vi "Sort_AI_Data.vi"(7 "Inclin":T3, 10 "AI_data":dbl[](array[numeric]), 11 "AlarmSettings":T1={"TC13"={"Enbl"=FALSE, "ErrsAndWarns"={0.0, 5.663716814159292, 7.168141592920354, 8.584070796460177}}, "AI1"={"Enbl"=FALSE, "ErrsAndWarns"={0.0, 5.663716814159292, 7.168141592920354, 8.584070796460177}}, "AI2"={"Enbl"=FALSE, "ErrsAndWarns"={0.0, 5.663716814159292, 7.168141592920354, 8.584070796460177}}, "AI3"={"Enbl"=FALSE, "ErrsAndWarns"={0.0, 5.663716814159292, 7.168141592920354, 8.584070796460177}}, "AI4"={"Enbl"=FALSE, "ErrsAndWarns"={0.0, 5.663716814159292, 7.168141592920354, 8.584070796460177}}, "AI5"={"Enbl"=FALSE, "ErrsAndWarns"={0.0, 5.663716814159292, 7.168141592920354, 8.584070796460177}}, "AI6"={"Enbl"=FALSE, "ErrsAndWarns"={0.0, 5.663716814159292, 7.168141592920354, 8.584070796460177}}, "AI18"={"Enbl"=FALSE, "ErrsAndWarns"={0.0, 5.663716814159292, 7.168141592920354, 8.584070796460177}}, "AI19"={"Enbl"=FALSE, "ErrsAndWarns"={0.0, 5.663716814159292, 7.168141592920354, 8.584070796460177}}, "TE1"={"Enbl"=FALSE, "ErrsAndWarns"={0.0, 5.663716814159292, 7.168141592920354, 8.584070796460177}}, "TE2"={"Enbl"=FALSE, "ErrsAndWarns"={0.0, 5.663716814159292, 7.168141592920354, 8.584070796460177}}, "TE3"={"Enbl"=FALSE, "ErrsAndWarns"={0.0, 5.663716814159292, 7.168141592920354, 8.584070796460177}}, "ADAM1"={"Enbl"=FALSE, "ErrsAndWarns"={0.0, 5.663716814159292, 7.168141592920354, 8.584070796460177}}, "ADAM2"={"Enbl"=FALSE, "ErrsAndWarns"={0.0, 5.663716814159292, 7.168141592920354, 8.584070796460177}}, "ADAM3"={"Enbl"=FALSE, "ErrsAndWarns"={0.0, 5.663716814159292, 7.168141592920354, 8.584070796460177}}, "ADAM4"={"Enbl"=FALSE, "ErrsAndWarns"={0.0, 5.663716814159292, 7.168141592920354, 8.584070796460177}}, "72CoBeacFreq"={"Enbl"=FALSE, "ErrsAndWarns"={0.0, 5.663716814159292, 7.168141592920354, 8.584070796460177}}, "72CoCalFreq"={"Enbl"=FALSE, "ErrsAndWarns"={0.0, 5.663716814159292, 7.168141592920354, 8.584070796460177}}, "84CoBeacFreq"={"Enbl"=FALSE, "ErrsAndWarns"={0.0, 5.663716814159292, 7.168141592920354, 8.584070796460177}}, "84CoCalFreq"={"Enbl"=FALSE, "ErrsAndWarns"={0.0, 5.663716814159292, 7.168141592920354, 8.584070796460177}}, "72Co_CalTonePwr"={"Enbl"=FALSE, "ErrsAndWarns"={0.0, 5.663716814159292, 7.168141592920354, 8.584070796460177}}, "72X_CalTonePwr"={"Enbl"=FALSE, "ErrsAndWarns"={0.0, 5.663716814159292, 7.168141592920354, 8.584070796460177}}, "84Co_CalTonePwr"={"Enbl"=FALSE, "ErrsAndWarns"={0.0, 5.663716814159292, 7.168141592920354, 8.584070796460177}}, "84X_CalTonePwr"={"Enbl"=FALSE, "ErrsAndWarns"={0.0, 5.663716814159292, 7.168141592920354, 8.584070796460177}}} {"84X_CalTonePwr"."ErrsAndWarns" scale=-120.0..-45.0; "72X_CalTonePwr"."ErrsAndWarns" scale=-120.0..-45.0; "84Co_CalTonePwr"."ErrsAndWarns" scale=-120.0..-45.0; "72Co_CalTonePwr"."ErrsAndWarns" scale=-120.0..-45.0; "84CoCalFreq"."ErrsAndWarns" scale=24.9..25.1; "84CoBeacFreq"."ErrsAndWarns" scale=25.5..27.0; "72CoCalFreq"."ErrsAndWarns" scale=24.9..25.1; "72CoBeacFreq"."ErrsAndWarns" scale=25.5..27.0; "ADAM4"."ErrsAndWarns" scale=30.0..52.0; "ADAM3"."ErrsAndWarns" scale=30.0..52.0; "ADAM2"."ErrsAndWarns" scale=30.0..52.0; "ADAM1"."ErrsAndWarns" scale=30.0..52.0; "TE3"."ErrsAndWarns" scale=30.0..52.0; "TE2"."ErrsAndWarns" scale=30.0..52.0; "TE1"."ErrsAndWarns" scale=20.0..52.0; "AI19"."ErrsAndWarns" scale=0.0..60.0; "AI18"."ErrsAndWarns" scale=-10.0..10.0; "AI6"."ErrsAndWarns" scale=0.0..35.0; "AI5"."ErrsAndWarns" scale=0.0..20.0; "AI4"."ErrsAndWarns" scale=0.0..15.0; "AI3"."ErrsAndWarns" scale=0.0..10.0; "AI2"."ErrsAndWarns" scale=0.0..10.0; "TC13"."ErrsAndWarns" scale=-10.0..40.0}) -> (2 "All_AI_Error_Status":T4, 3 "AI_Variant":variant)   [LabVIEW 2018]
uses:
  Controls/Clusts/All_AI_Error_Status.ctl
  Controls/Clusts/ErrorStatus.ctl
  Controls/Clusts/Inclinometer_User_Cfg.ctl
  Controls/Clusts/AlarmSettingsClust.ctl
  Controls/Clusts/AlarmThresh_OneChan.ctl
  Controls/Clusts/AI_Clust.ctl
  Controls/Clusts/All_AI_Error_and_Data.ctl
  Controls/Enums/Inclinometer_Direction.ctl
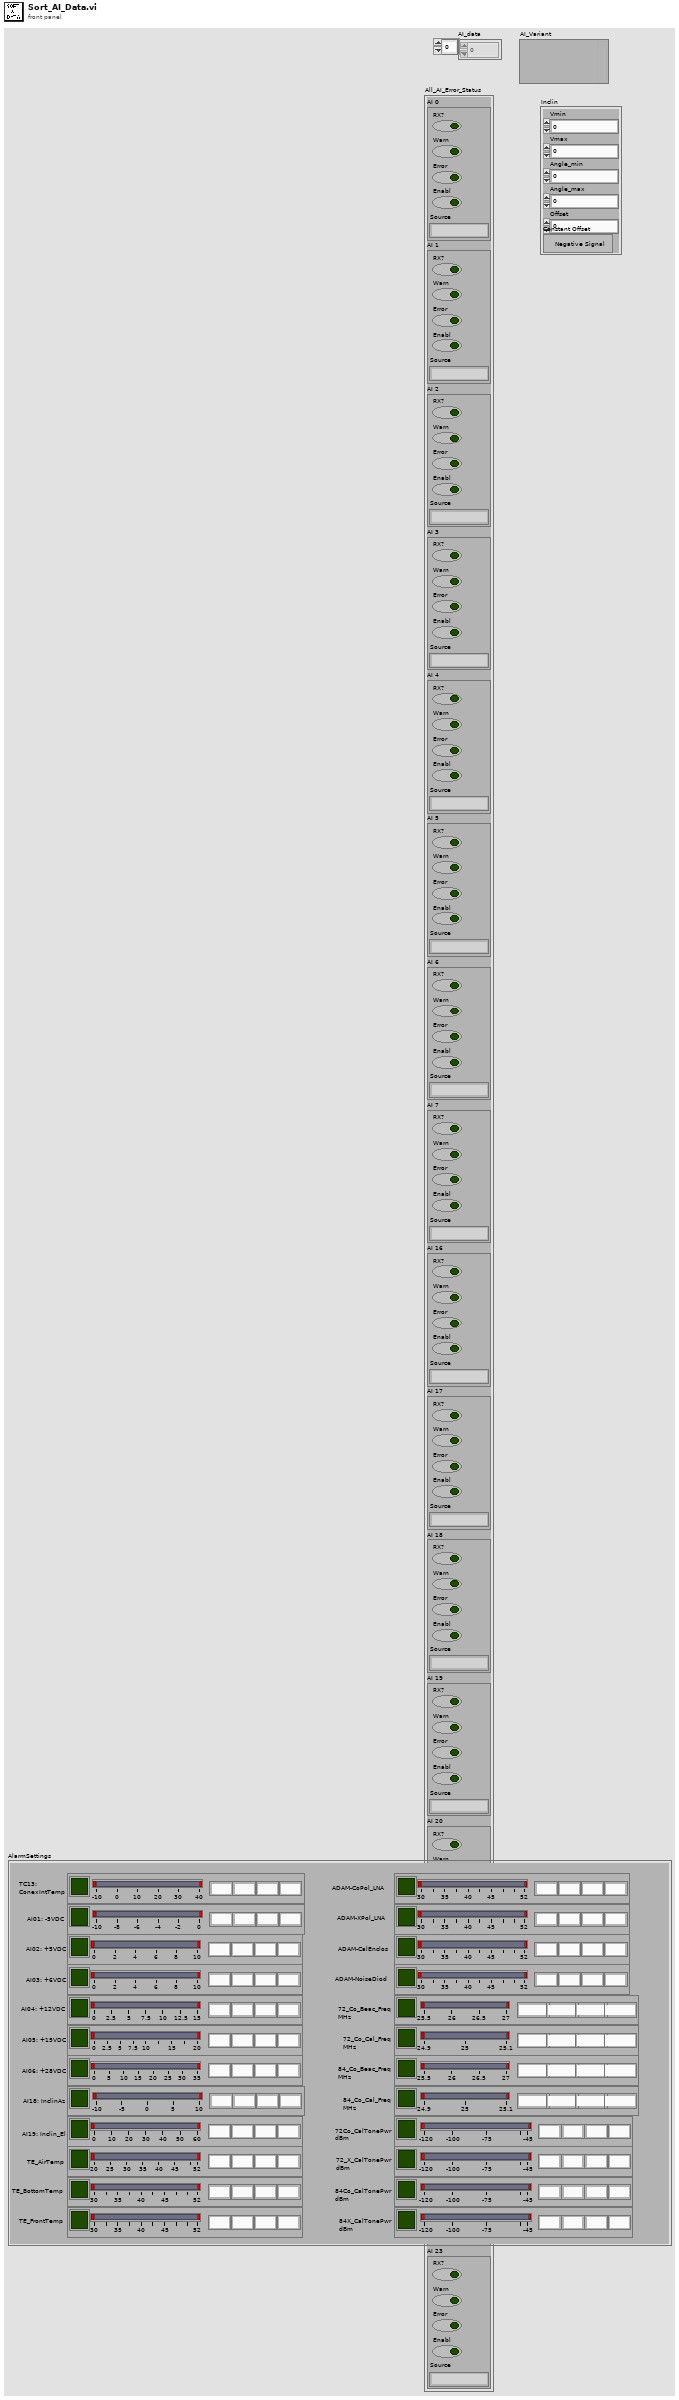
[diagram p1: front panel]
types:
  T1 = typedef "AlarmSettingsClust.ctl" = cluster{"TC13":T2, "AI1":T2, "AI2":T2, "AI3":T2, "AI4":T2, "AI5":T2, "AI6":T2, "AI18":T2, "AI19":T2, "TE1":T2, "TE2":T2, "TE3":T2, "ADAM1":T2, "ADAM2":T2, "ADAM3":T2, "ADAM4":T2, "72CoBeacFreq":T2, "72CoCalFreq":T2, "84CoBeacFreq":T2, "84CoCalFreq":T2, "72Co_CalTonePwr":T2, "72X_CalTonePwr":T2, "84Co_CalTonePwr":T2, "84X_CalTonePwr":T2}
  T2 = typedef "AlarmThresh_OneChan.ctl" = cluster{"Enbl":bool, "ErrsAndWarns":cluster{dbl, dbl, dbl, dbl}}
  T3 = typedef "Inclinometer_User_Cfg.ctl" = cluster{"Vmin":dbl, "Vmax":dbl, "Angle_min":dbl, "Angle_max":dbl, "Offset":dbl, "Pos_Neg":bool}
  T4 = typedef "All_AI_Error_Status.ctl" = cluster{"AI 0":T5, "AI 1":T5, "AI 2":T5, "AI 3":T5, "AI 4":T5, "AI 5":T5, "AI 6":T5, "AI 7":T5, "AI 16":T5, "AI 17":T5, "AI 18":T5, "AI 19":T5, "AI 20":T5, "AI 21":T5, "AI 22":T5, "AI 23":T5}
  T5 = typedef "ErrorStatus.ctl" = cluster{"RX?":bool, "Warn":bool, "Error":bool, "Enabl":bool, "Source":string}
  T6 = typedef "Inclinometer_Direction.ctl" = enum16{"Elev", "Azim"}
  T7 = typedef "All_AI_Error_and_Data.ctl" = cluster{"AI":T8, "AllErrorStatus":T4}
  T8 = typedef "AI_Clust.ctl" = cluster{"TimeString":string, "Time Stamp":dbl, "AI0_Unused":dbl, "AI1_-5V":dbl, "AI2_+5V":dbl, "AI3_+6V":dbl, "AI4_+12V":dbl, "AI5_+15V":dbl, "AI6_+28V":dbl, "AI7_Unused":dbl, "Ai16_72GHz_CalPower":dbl, "Ai17_84GHz_CalPower":dbl, "Ai18_InclinAz":dbl, "Ai19_InclinEl":dbl, "Ai20_BlowerPwr":dbl, "Ai21_Unused":dbl, "Ai22_Unused":dbl, "Ai23_Unused":dbl, "InclinA_StdDev":dbl, "InclinB_StdDev":dbl, "InclinAz_Unfilt":dbl, "InclinEl_Unfilt":dbl}
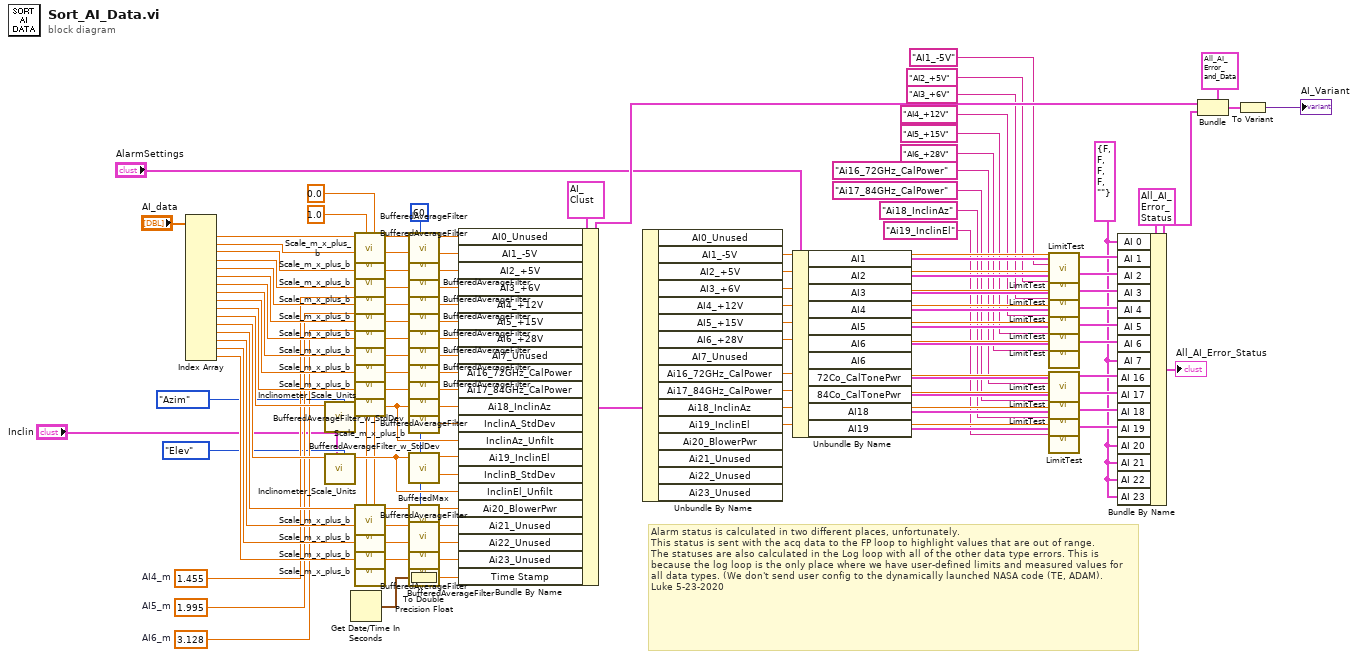
[diagram p0: block diagram]
diagram:
  w19 = T5 {"RX?"=FALSE, "Warn"=FALSE, "Error"=FALSE, "Enabl"=FALSE, "Source"=""} ("AI 0")
  w25 = 3.128  # AI6_m
  w26 = 1.995  # AI5_m
  w27 = 1.455  # AI4_m
  w24 = 0.0 ("b")
  w23 = 1.0 ("m")
  w13 = 60 ("dimension size")
  # "Alarm status is calculated in two different places, unfortunately.\nThis status is sent with the acq data to the FP loop to highlight values that are out of range.\nThe statuses are also calculated in the Log loop with all of the other data type errors. This is because the log loop is the only place where we have user-defined limits and measured values for all data types. (We don't send user config to the dynamically launched NASA code (TE, ADAM). \nLuke 5-23-2020"
  n1 = Index Array(array="AI_data") -> (element #1=w54:dbl, element #2=w52:dbl, element #3=w51:dbl, element #4=w50:dbl, element #5=w49:dbl, element #6=w48:dbl, element #7=w47:dbl, element #8=w46:dbl, element #9=w45:dbl, element #10=w44:dbl, element #11=w62:dbl, element #12=w61:dbl, element #13=w43:dbl, element #14=w42:dbl, element #15=w41:dbl, element #16=w40:dbl)  [unwired: 16 in]
  n2 = call "Inclinometer_Scale_Units.vi"("Enum"=Inclinometer_Direction."Azim", "Inclin"="Inclin", "Unscaled"=w62) -> ("Scaled"=w56:dbl)  [unwired: 8 in]
  n3 = call "Inclinometer_Scale_Units.vi"("Enum"=Inclinometer_Direction."Elev", "Inclin"="Inclin", "Unscaled"=w61) -> ("Scaled"=w55:dbl)  [unwired: 8 in]
  n4 = Get Date/Time In Seconds() -> (seconds since 1Jan1904=w1:timestamp)
  n5 = call "Scale_m_x_plus_b.vi"("b"=w24, "m"=w23, "Signal"=w54) -> ("Scaled Signal"=w53:dbl)  [unwired: 8 in]
  n6 = call "Scale_m_x_plus_b.vi"("b"=w24, "m"=w23, "Signal"=w52) -> ("Scaled Signal"=w39:dbl)  [unwired: 8 in]
  n7 = call "Scale_m_x_plus_b.vi"("b"=w24, "m"=w23, "Signal"=w51) -> ("Scaled Signal"=w38:dbl)  [unwired: 8 in]
  n8 = call "Scale_m_x_plus_b.vi"("b"=w24, "m"=w23, "Signal"=w50) -> ("Scaled Signal"=w37:dbl)  [unwired: 8 in]
  n9 = call "Scale_m_x_plus_b.vi"("b"=w24, "m"=w27, "Signal"=w49) -> ("Scaled Signal"=w36:dbl)  [unwired: 8 in]
  n10 = call "Scale_m_x_plus_b.vi"("b"=w24, "m"=w26, "Signal"=w48) -> ("Scaled Signal"=w35:dbl)  [unwired: 8 in]
  n11 = call "Scale_m_x_plus_b.vi"("b"=w24, "m"=w25, "Signal"=w47) -> ("Scaled Signal"=w34:dbl)  [unwired: 8 in]
  n12 = call "Scale_m_x_plus_b.vi"("b"=w24, "m"=w23, "Signal"=w46) -> ("Scaled Signal"=w33:dbl)  [unwired: 8 in]
  n13 = call "Scale_m_x_plus_b.vi"("b"=w24, "m"=w23, "Signal"=w45) -> ("Scaled Signal"=w32:dbl)  [unwired: 8 in]
  n14 = call "Scale_m_x_plus_b.vi"("b"=w24, "m"=w23, "Signal"=w44) -> ("Scaled Signal"=w31:dbl)  [unwired: 8 in]
  n15 = call "Scale_m_x_plus_b.vi"("b"=w24, "m"=w23, "Signal"=w43) -> ("Scaled Signal"=w15:dbl)  [unwired: 8 in]
  n16 = call "Scale_m_x_plus_b.vi"("b"=w24, "m"=w23, "Signal"=w42) -> ("Scaled Signal"=w30:dbl)  [unwired: 8 in]
  n17 = call "Scale_m_x_plus_b.vi"("b"=w24, "m"=w23, "Signal"=w41) -> ("Scaled Signal"=w29:dbl)  [unwired: 8 in]
  n18 = call "Scale_m_x_plus_b.vi"("b"=w24, "m"=w23, "Signal"=w40) -> ("Scaled Signal"=w28:dbl)  [unwired: 8 in]
  n19 = call "BufferedAverageFilter.vi"("Buffer Size"=w13, "Signal"=w53) -> ("FilteredSignal"=w75:dbl)  [unwired: 9 in]
  n20 = call "BufferedAverageFilter.vi"("Buffer Size"=w13, "Signal"=w39) -> ("FilteredSignal"=w74:dbl)  [unwired: 9 in]
  n21 = call "BufferedAverageFilter.vi"("Buffer Size"=w13, "Signal"=w38) -> ("FilteredSignal"=w73:dbl)  [unwired: 9 in]
  n22 = call "BufferedAverageFilter.vi"("Buffer Size"=w13, "Signal"=w37) -> ("FilteredSignal"=w72:dbl)  [unwired: 9 in]
  n23 = call "BufferedAverageFilter.vi"("Buffer Size"=w13, "Signal"=w36) -> ("FilteredSignal"=w71:dbl)  [unwired: 9 in]
  n24 = call "BufferedAverageFilter.vi"("Buffer Size"=w13, "Signal"=w35) -> ("FilteredSignal"=w70:dbl)  [unwired: 9 in]
  n25 = call "BufferedAverageFilter.vi"("Buffer Size"=w13, "Signal"=w34) -> ("FilteredSignal"=w69:dbl)  [unwired: 9 in]
  n26 = call "BufferedAverageFilter.vi"("Buffer Size"=w13, "Signal"=w33) -> ("FilteredSignal"=w68:dbl)  [unwired: 9 in]
  n27 = call "BufferedAverageFilter.vi"("Buffer Size"=w13, "Signal"=w32) -> ("FilteredSignal"=w67:dbl)  [unwired: 9 in]
  n28 = call "BufferedAverageFilter.vi"("Buffer Size"=w13, "Signal"=w31) -> ("FilteredSignal"=w66:dbl)  [unwired: 9 in]
  n29 = call "BufferedAverageFilter_w_StdDev.vi"("Buffer Size"=w13, "Signal"=w56) -> ("FilteredSignal"=w60:dbl, "standard deviation"=w58:dbl)  [unwired: 8 in]
  n30 = call "BufferedAverageFilter_w_StdDev.vi"("Buffer Size"=w13, "Signal"=w55) -> ("FilteredSignal"=w59:dbl, "standard deviation"=w57:dbl)  [unwired: 8 in]
  n31 = call "BufferedMax.vi"("Buffer Size"=w13, "Signal"=w15) -> ("MaxValue"=w14:dbl)  [unwired: 9 in]
  n32 = call "BufferedAverageFilter.vi"("Buffer Size"=w13, "Signal"=w30) -> ("FilteredSignal"=w65:dbl)  [unwired: 9 in]
  n33 = call "BufferedAverageFilter.vi"("Buffer Size"=w13, "Signal"=w29) -> ("FilteredSignal"=w64:dbl)  [unwired: 9 in]
  n34 = call "BufferedAverageFilter.vi"("Buffer Size"=w13, "Signal"=w28) -> ("FilteredSignal"=w63:dbl)  [unwired: 9 in]
  n35 = To Double Precision Float(number=w1) -> (double precision float=w2:dbl)
  n36 = Bundle By Name(cluster=T8 {"TimeString"="", "Time Stamp"=0.0, "AI0_Unused"=0.0, "AI1_-5V"=0.0, "AI2_+5V"=0.0, "AI3_+6V"=0.0, "AI4_+12V"=0.0, "AI5_+15V"=0.0, "AI6_+28V"=0.0, "AI7_Unused"=0.0, "Ai16_72GHz_CalPower"=0.0, "Ai17_84GHz_CalPower"=0.0, "Ai18_InclinAz"=0.0, "Ai19_InclinEl"=0.0, "Ai20_BlowerPwr"=0.0, "Ai21_Unused"=0.0, "Ai22_Unused"=0.0, "Ai23_Unused"=0.0, "InclinA_StdDev"=0.0, "InclinB_StdDev"=0.0, "InclinAz_Unfilt"=0.0, "InclinEl_Unfilt"=0.0} ("AI"), "AI0_Unused"=w75, "AI1_-5V"=w74, "AI2_+5V"=w73, "AI3_+6V"=w72, "AI4_+12V"=w71, "AI5_+15V"=w70, "AI6_+28V"=w69, "AI7_Unused"=w68, "Ai16_72GHz_CalPower"=w67, "Ai17_84GHz_CalPower"=w66, "Ai18_InclinAz"=w60, "InclinA_StdDev"=w58, "InclinAz_Unfilt"=w56, "Ai19_InclinEl"=w59, "InclinB_StdDev"=w57, "InclinEl_Unfilt"=w55, "Ai20_BlowerPwr"=w14, "Ai21_Unused"=w65, "Ai22_Unused"=w64, "Ai23_Unused"=w63, "Time Stamp"=w2) -> (w79:T8)
  n37 = Unbundle By Name(w79) -> ("AI1_-5V"=w108:dbl, "AI2_+5V"=w107:dbl, "AI3_+6V"=w105:dbl, "AI4_+12V"=w104:dbl, "AI5_+15V"=w103:dbl, "AI6_+28V"=w102:dbl, "Ai16_72GHz_CalPower"=w101:dbl, "Ai17_84GHz_CalPower"=w100:dbl, "Ai18_InclinAz"=w17:dbl, "Ai19_InclinEl"=w16:dbl)  [unwired: 6 out]
  n38 = Unbundle By Name("AlarmSettings") -> ("AI1"=w106:T2, "AI2"=w99:T2, "AI3"=w98:T2, "AI4"=w97:T2, "AI5"=w96:T2, "AI6"=w95:T2, "72Co_CalTonePwr"=w94:T2, "84Co_CalTonePwr"=w93:T2, "AI18"=w92:T2, "AI19"=w91:T2)  [unwired: 1 out]
  n39 = call "LimitTest.vi"("AlarmCfg"=w106, "Source"="AI1_-5V", "Data"=w108) -> ("ErrorStatus"=w89:T5)  [unwired: 8 in]
  n40 = call "LimitTest.vi"("AlarmCfg"=w99, "Source"="AI2_+5V", "Data"=w107) -> ("ErrorStatus"=w88:T5)  [unwired: 8 in]
  n41 = call "LimitTest.vi"("AlarmCfg"=w98, "Source"="AI3_+6V", "Data"=w105) -> ("ErrorStatus"=w87:T5)  [unwired: 8 in]
  n42 = call "LimitTest.vi"("AlarmCfg"=w97, "Source"="AI4_+12V", "Data"=w104) -> ("ErrorStatus"=w86:T5)  [unwired: 8 in]
  n43 = call "LimitTest.vi"("AlarmCfg"=w96, "Source"="AI5_+15V", "Data"=w103) -> ("ErrorStatus"=w85:T5)  [unwired: 8 in]
  n44 = call "LimitTest.vi"("AlarmCfg"=w95, "Source"="AI6_+28V", "Data"=w102) -> ("ErrorStatus"=w84:T5)  [unwired: 8 in]
  n45 = call "LimitTest.vi"("AlarmCfg"=w94, "Source"="Ai16_72GHz_CalPower", "Data"=w101) -> ("ErrorStatus"=w83:T5)  [unwired: 8 in]
  n46 = call "LimitTest.vi"("AlarmCfg"=w93, "Source"="Ai17_84GHz_CalPower", "Data"=w100) -> ("ErrorStatus"=w82:T5)  [unwired: 8 in]
  n47 = call "LimitTest.vi"("AlarmCfg"=w92, "Source"="Ai18_InclinAz", "Data"=w17) -> ("ErrorStatus"=w81:T5)  [unwired: 8 in]
  n48 = call "LimitTest.vi"("AlarmCfg"=w91, "Source"="Ai19_InclinEl", "Data"=w16) -> ("ErrorStatus"=w80:T5)  [unwired: 8 in]
  n49 = Bundle By Name(cluster=T4 {"AI 0"={"RX?"=FALSE, "Warn"=FALSE, "Error"=FALSE, "Enabl"=FALSE, "Source"=""}, "AI 1"={"RX?"=FALSE, "Warn"=FALSE, "Error"=FALSE, "Enabl"=FALSE, "Source"=""}, "AI 2"={"RX?"=FALSE, "Warn"=FALSE, "Error"=FALSE, "Enabl"=FALSE, "Source"=""}, "AI 3"={"RX?"=FALSE, "Warn"=FALSE, "Error"=FALSE, "Enabl"=FALSE, "Source"=""}, "AI 4"={"RX?"=FALSE, "Warn"=FALSE, "Error"=FALSE, "Enabl"=FALSE, "Source"=""}, "AI 5"={"RX?"=FALSE, "Warn"=FALSE, "Error"=FALSE, "Enabl"=FALSE, "Source"=""}, "AI 6"={"RX?"=FALSE, "Warn"=FALSE, "Error"=FALSE, "Enabl"=FALSE, "Source"=""}, "AI 7"={"RX?"=FALSE, "Warn"=FALSE, "Error"=FALSE, "Enabl"=FALSE, "Source"=""}, "AI 16"={"RX?"=FALSE, "Warn"=FALSE, "Error"=FALSE, "Enabl"=FALSE, "Source"=""}, "AI 17"={"RX?"=FALSE, "Warn"=FALSE, "Error"=FALSE, "Enabl"=FALSE, "Source"=""}, "AI 18"={"RX?"=FALSE, "Warn"=FALSE, "Error"=FALSE, "Enabl"=FALSE, "Source"=""}, "AI 19"={"RX?"=FALSE, "Warn"=FALSE, "Error"=FALSE, "Enabl"=FALSE, "Source"=""}, "AI 20"={"RX?"=FALSE, "Warn"=FALSE, "Error"=FALSE, "Enabl"=FALSE, "Source"=""}, "AI 21"={"RX?"=FALSE, "Warn"=FALSE, "Error"=FALSE, "Enabl"=FALSE, "Source"=""}, "AI 22"={"RX?"=FALSE, "Warn"=FALSE, "Error"=FALSE, "Enabl"=FALSE, "Source"=""}, "AI 23"={"RX?"=FALSE, "Warn"=FALSE, "Error"=FALSE, "Enabl"=FALSE, "Source"=""}} ("AllErrorStatus"), "AI 0"=w19, "AI 1"=w89, "AI 2"=w88, "AI 3"=w87, "AI 4"=w86, "AI 5"=w85, "AI 6"=w84, "AI 7"=w19, "AI 16"=w83, "AI 17"=w82, "AI 18"=w81, "AI 19"=w80, "AI 20"=w19, "AI 21"=w19, "AI 22"=w19, "AI 23"=w19) -> (w77:T4)
  "All_AI_Error_Status" <- w77
  n50 = Bundle(cluster=T7 {"AI"={"TimeString"="", "Time Stamp"=0.0, "AI0_Unused"=0.0, "AI1_-5V"=0.0, "AI2_+5V"=0.0, "AI3_+6V"=0.0, "AI4_+12V"=0.0, "AI5_+15V"=0.0, "AI6_+28V"=0.0, "AI7_Unused"=0.0, "Ai16_72GHz_CalPower"=0.0, "Ai17_84GHz_CalPower"=0.0, "Ai18_InclinAz"=0.0, "Ai19_InclinEl"=0.0, "Ai20_BlowerPwr"=0.0, "Ai21_Unused"=0.0, "Ai22_Unused"=0.0, "Ai23_Unused"=0.0, "InclinA_StdDev"=0.0, "InclinB_StdDev"=0.0, "InclinAz_Unfilt"=0.0, "InclinEl_Unfilt"=0.0}, "AllErrorStatus"={"AI 0"={"RX?"=FALSE, "Warn"=FALSE, "Error"=FALSE, "Enabl"=FALSE, "Source"=""}, "AI 1"={"RX?"=FALSE, "Warn"=FALSE, "Error"=FALSE, "Enabl"=FALSE, "Source"=""}, "AI 2"={"RX?"=FALSE, "Warn"=FALSE, "Error"=FALSE, "Enabl"=FALSE, "Source"=""}, "AI 3"={"RX?"=FALSE, "Warn"=FALSE, "Error"=FALSE, "Enabl"=FALSE, "Source"=""}, "AI 4"={"RX?"=FALSE, "Warn"=FALSE, "Error"=FALSE, "Enabl"=FALSE, "Source"=""}, "AI 5"={"RX?"=FALSE, "Warn"=FALSE, "Error"=FALSE, "Enabl"=FALSE, "Source"=""}, "AI 6"={"RX?"=FALSE, "Warn"=FALSE, "Error"=FALSE, "Enabl"=FALSE, "Source"=""}, "AI 7"={"RX?"=FALSE, "Warn"=FALSE, "Error"=FALSE, "Enabl"=FALSE, "Source"=""}, "AI 16"={"RX?"=FALSE, "Warn"=FALSE, "Error"=FALSE, "Enabl"=FALSE, "Source"=""}, "AI 17"={"RX?"=FALSE, "Warn"=FALSE, "Error"=FALSE, "Enabl"=FALSE, "Source"=""}, "AI 18"={"RX?"=FALSE, "Warn"=FALSE, "Error"=FALSE, "Enabl"=FALSE, "Source"=""}, "AI 19"={"RX?"=FALSE, "Warn"=FALSE, "Error"=FALSE, "Enabl"=FALSE, "Source"=""}, "AI 20"={"RX?"=FALSE, "Warn"=FALSE, "Error"=FALSE, "Enabl"=FALSE, "Source"=""}, "AI 21"={"RX?"=FALSE, "Warn"=FALSE, "Error"=FALSE, "Enabl"=FALSE, "Source"=""}, "AI 22"={"RX?"=FALSE, "Warn"=FALSE, "Error"=FALSE, "Enabl"=FALSE, "Source"=""}, "AI 23"={"RX?"=FALSE, "Warn"=FALSE, "Error"=FALSE, "Enabl"=FALSE, "Source"=""}}}, "AI"=w79, "AllErrorStatus"=w77) -> (w78:T7)
  n51 = To Variant(anything=w78) -> (Variant=→"AI_Variant":variant)
